vi "S2C_M2p5942_Proc_Close.vi"(8 "Error In":errorcluster) -> (0 "Error Out":errorcluster)   [LabVIEW 2024]
uses:
  S2C_M2p5942_Proc_Globals.vi
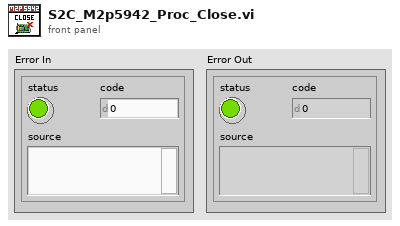
[diagram p1: front panel]
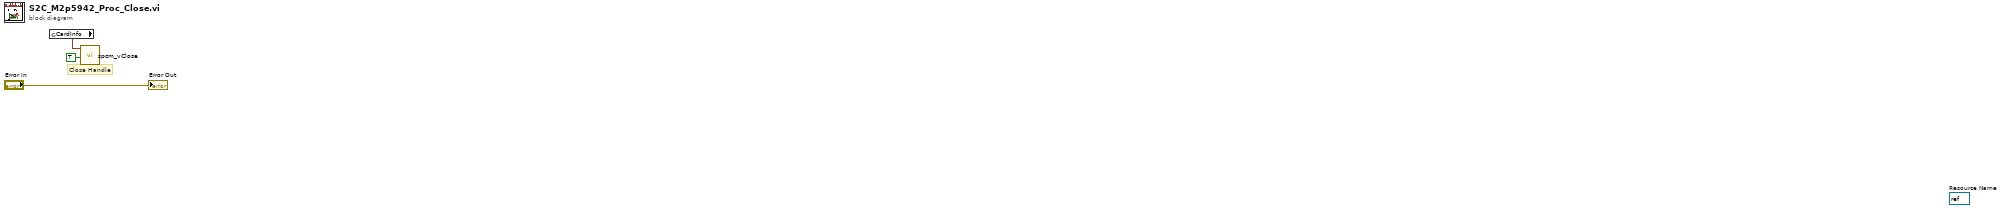
[diagram p0: block diagram]
diagram:
  (unwired) refnum<visa-resource-name> refnum  # Resource Name
  # "Close Handle"
  n1 = global read "S2C_M2p5942_Proc_Globals.vi" "CardInfo"() -> (w3:cluster{"Card Handle":u64, "Error Code":u32})
  n2 = call "spcm_vClose.vi"("Free All Devices"=TRUE, "Card Info In"=w3) -> ()  [unwired: 6 in]
  "Error Out" <- "Error In"
